vi "AlliGator Phasor Ratio Actions.vi"(0 "AlliGator Q Elements in":T4[](array[typedef]), 1 "VI in":refnum<vi>, 2 "Script in":bool, 5 "data value reference in":refnum<data-value>, 7 "AlliGator Q Event in":T5=enum."GUI:Idle", 9 "Data":variant, 11 "error in (no error)":errorcluster, 12 "AlliGator Ctrl Refnums":T6) -> (3 "Script out":bool, 4 "AlliGator Q Elements out":T4[](array[typedef]), 6 "Data Value Reference out":refnum<data-value>, 10 "[Notebook Message]":T1[](array[typedef]) {"Message Style"."Text Alignment" items=["Left", "Right", "Center"]}, 15 "error out":errorcluster)   [LabVIEW 2021, in "AlliGator Action Engine.lvlib"]
doc: "Processes AlliGator phasor ratio-related actions."
uses:
  AlliGator Action Engine.lvlib
  AlliGator Internal Variables v2.ctl
  <vilib>/vision/Image Controls.llb/IMAQ Image.ctl
  AlliGator Gate Image Set.ctl
  AlliGator FLI Dataset Type.ctl
  AlliGator Data Series Type.ctl
  AlliGator Dataset Channel.ctl
  AlliGator Gate Arithmetic.ctl
  AlliGator Displayed Image.ctl
  Image/Named ROI Description.ctl
  AlliGator Decay Metadata v3.ctl
  AlliGator Decay Background Subtraction Info.ctl
  AlliGator Baseline Subtraction Method.ctl
  Graphs/XY Graph/XY Graph Plot Shift Parameters.ctl
  Graphs/XY Graph/XY Graph Plot Shift Method.ctl
  AlliGator Decay Extrapolation Parameters.ctl
  Phasor/Calibration Phasor (m, phi).ctl
  Phasor/Phasor Reference Series.ctl
  Phasor/Phasor Calibration Map v2.ctl
  Phasor/Phasor (g, s).ctl
  AlliGator Raw Phasor Plot Data v4.ctl
  Phasor/Phasor Standard Deviation Options.ctl
  AlliGator Phasor Multi-Harmonic Data.ctl
  Phasor/Phasor Harmonic Data.ctl
  AlliGator Decay Fit Options & Parameters v2.ctl
  Fits/IRF(X)PSED/Decay Fit Options v2.ctl
  Fits/Decay Convolution/Decay Model.ctl
  Fits/Residual Type.ctl
  Fits/IRF(X)PSED/Fit Weights Type.ctl
  Fits/Non-linear Fitting Method v2.ctl
  Fits/Fit Calculation Method.ctl
  Fits/Non-linear Fitting Algorithm.ctl
  AlliGator Decay Fit Parameter Constraints 2.ctl
  Fits/IRF(X)PSED/Decay Fit Parameters In List.ctl
  Fits/IRF(X)PSED/MLE Baseline Offset Type.ctl
  AlliGator Decay Preprocessing Parameters.ctl
  Fits/IRF(X)PSED/Decay Fit Parameters & Derived Quantities List.ctl
  AlliGator Q Event.ctl
  AlliGator Ctrl Refnums.ctl
  AlliGator Other Ctrl Refnums.ctl
  AlliGator State Indicator.ctl
  AlliGator Phasor Plot Ctrl Refnums.ctl
  AlliGator Phasor Graph Ctrl Refnums.ctl
  Phasor/Phasor Calibration Type.ctl
  AlliGator Dataset Ctrl Refnums.ctl
  AlliGator Registered Events Ctrl Refnums.ctl
  AlliGator Image Histogram Control Refnums.ctl
  Histograms/Linear Histogram Options.ctl
  Histograms/Histogram Bin Option.ctl
  Histograms/Histogram Bin Position.ctl
  AlliGator Decay Fit Map Control Refnums.ctl
  AlliGator Q Element.ctl
  Notebook/Notebook Message Object.ctl
  Rich Text Box/Text Formatting.ctl
  Rich Text Box/Text Colors.ctl
  AlliGator Phasor Ratio at Mouse Location Data.ctl
  Graphs/XY Graph/XY Graph Mouse Click Event Data.ctl
  Graphs/XY Graph/XY Graph Refnum.ctl
  <vilib>/Utility/miscctls.llb/LVPoint32TypeDef.ctl
  AlliGator Phasor Reference Data.ctl
  Alligator Elements Order in Action Stack.ctl
  AlliGator State Indicators List.ctl
  AlliGator Variables List.ctl
  Variant/Variant to Data/Variant to I32.vi
  Graphs/Get Plot at Mouse Click (XY Graph)/Get Plot at Mouse Click [AAC].vi
  Variant/Variant to Data/Variant to Boolean.vi
  Variant/Variant to Data/Variant to Path.vi
  AlliGator Add Single Action to Stack.vi
  Variant/Variant to Data/Variant to DBL.vi
  Variant/Variant to Data/Variant to Data.lvlib
  GUI/GUI.lvlib
  AlliGator Source Image.lvlib
  AlliGator Phasor Graph.lvlib
  AlliGator Phasor Ratio.lvlib
  Rich Text Box/Rich Text Box.lvlib
  AlliGator Internal Variables.lvlib
  Graphs/XY Graph/XY Graph Add-Ons.lvlib
  Graphs/Graphs.lvlib
  AlliGator Globals, Variables & Constants.lvlib
  AlliGator GUI.lvlib
  AlliGator Settings.lvlib
  AlliGator Phasor Calibration.lvlib
  Notebook/Notebook.lvlib
  Phasor/Phasor.lvlib
  Image/Image.lvlib
  AlliGator Decay Preprocessing.lvlib
  AlliGator Files.lvlib
  AlliGator Phasor Plot.lvlib
  Fits/Fits.lvlib
  AlliGator Decay Fit.lvlib
  AlliGator Decay Fit Parameter Map.lvlib
  AlliGator Dual-Channel Datasets.lvlib
  Histograms/Histogram Window.lvlib
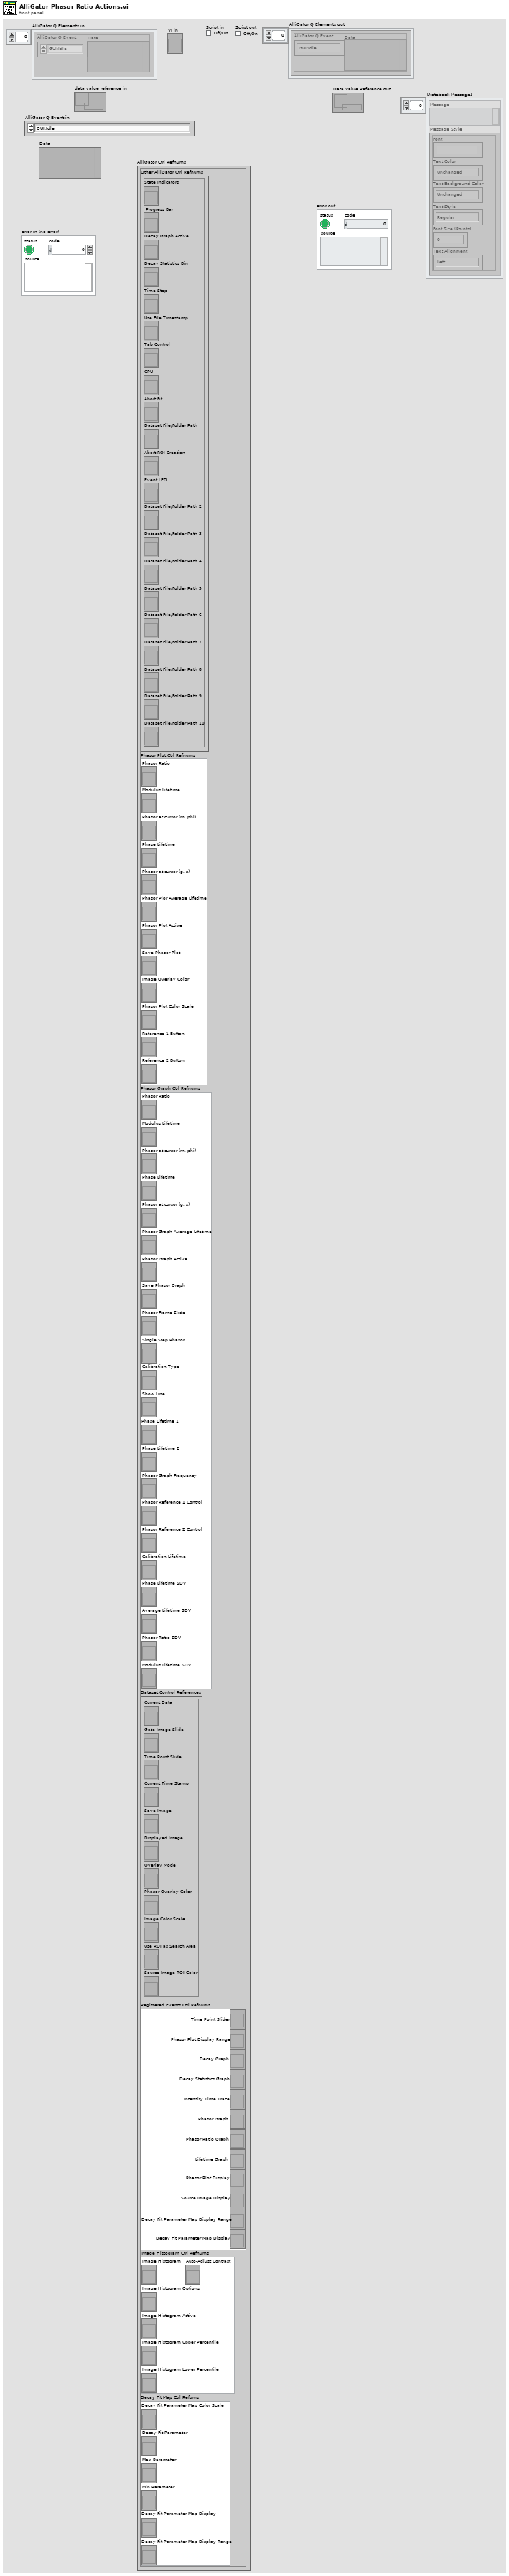
[diagram p1: front panel]
types:
  T1 = typedef "Notebook.lvlib/Notebook Message Object.ctl" = cluster{"Message":string, "Message Style":T2}
  T2 = typedef "Rich Text Box.lvlib/Text Formatting.ctl" = cluster{"Font":string, "Text Color":T3, "Text Background Color":T3, "Text Style":enum16{"Regular", "Bold", "Italic", "Underline", "Strikeout"}, "Font Size (Points)":dbl, "Text Alignment":i32}
  T3 = typedef "Rich Text Box.lvlib/Text Colors.ctl" = enum16{"Unchanged", "Black", "Blue", "Brown", "Gray", "Green", "Orange", "Pink", "Red", "White"}
  T4 = typedef "AlliGator Action Engine.lvlib/AlliGator Q Element.ctl" = cluster{"AlliGator Q Event":T5, "Data":variant}
  T5 = typedef "AlliGator Action Engine.lvlib/AlliGator Q Event.ctl" = enum16{"---- Files ----", "Files:Set Batch Export Files To Save", "Files:Set Dataset Loading & Pre-processing Options", "Files:Check #Frames in Dataset", "Files:Increment Frame Index", "Files:Open Mask Image", "Files:Open White Light Image", "Files:Open Single Dataset", "Files:New Folder of Folders Selected", "Files:Load File (all Types)_Scriptable", "Files:Move Flattened Series to Folders Series", "Files:Select Folder", "Files:Load FLI Dataset", "Files:Load Swiss SPAD 1 Dataset", "Files:Load Swiss SPAD 2 Dataset", "Files:Load .sdt FLI Dataset", "Files:Load .ptu FLI Dataset", "Files:Load .bin FLI Dataset", "Files:Load Single Gate Image Folder", "Files:Load I/m/phi Dataset (deprecated)", "Files:Load Single Image", "Files:Subtract Background File", "Files:Export FLI Dataset", "Files:Load HDF5 FLI Dataset", "Files:Set Destination File Path", "Files:Save Mask Image", "Files:Batch Conversion", "Files:New Folder Selected", "Files:Close FLI Dataset", "Files:Close FLI Dataset Series", "Files:Close White Light Image", "Files:Close Mask Image", "---- FLI Dataset ----", "FLI Dataset:Channel Arithmetic", "FLI Dataset:Export Average Lifetime Map as ASCII", "FLI Dataset:Export User-Defined Quantity Map as ASCII", "FLI Dataset:Python Function FLI Dataset Event", "FLI Dataset:ROI Analysis", "FLI Dataset:Tilted Logistic Square Gated IRF Characteristics Map", "FLI Dataset:Logistic Square Gated IRF Characteristics Map", "FLI Dataset:Square Gated IRF Characteristics Map", "FLI Dataset:Multi-ROI Single-Pixel Phasor Analysis", "FLI Dataset:Multi-ROI Single-Pixel NLSF Analysis", "FLI Dataset:All ROIs IRF Extraction", "FLI Dataset:All ROIs Decay Fit Non-Interactive (Fast + Individual IRF)", "FLI Dataset:All ROIs Phasor Analysis", "FLI Dataset:All ROIs Decay Fit", "FLI Dataset:Fluorescence Decay Statistics", "FLI Dataset:Update Decay Statistics Graph", "FLI Dataset:Get Decay from ROI", "FLI Dataset:All ROIs Average Lifetimes", "---- FLI Dataset Series ----", "FLI Dataset Series:Sum All Datasets in Series", "FLI Dataset Series:Add Dataset to Accumulated Dataset", "FLI Dataset Series:Display Accumulated Dataset", "FLI Dataset Series:Clear Dataset Series Sum", "FLI Dataset Series:Time-Series Analysis (NLSF)", "FLI Dataset Series:Time-Series Analysis (Phasor)", "---- Image ----", "Image:Update Image Profile Plots", "Image:Image Histogram Cursor Move", "Image:Image Histogram", "Image:Image Contrast", "Image:Set Image Histogram Cursor Move Flag", "Image:Clear Image Overlay", "Image:Use ROI as Search Area", "Image:Set ROI Diameter", "Image:Save Image Data as TIFF", "Image:Save Displayed Image with Overlay", "Image:Save Image Overlay Only", "Image:Save Image as Hot Pixel Mask", "Image:Change Source Image Color Palette", "Image:Copy Image to Clipboard", "Image:Source Image ROI Selection", "Image:Delete All ROIs", "Image:Delete All Unselected ROIs", "Image:Delete ROI", "Image:Merge All ROIs", "Image:Store ROI", "Image:Source Image ROI Storage", "Image:Export ROI Description to Notebook", "Image:Save ROI", "Image:Load ROI", "Image:Paste ROI Definition", "Image:Clear ROI", "Image:Identify ROIs in Mask Image", "Image:Create Complementary ROI", "Image:Create Contour ROI", "Image:Create ROI(s) from Pixels with Peak above Min_Scriptable", "Image:Create ROI(s) from Pixels with Intensity above Min_Scriptable", "Image:Compute ROI Statistics", "Image:Delete ROI(s) based on ROI Characteristics", "Image:Create ROI Grid", "Image:ROI to Individual Pixel ROIs", "Image:Python Function Source Image Event", "Image:Show Phasor Calibration Map ROI Centers", "Image:Convert ROI to Mask Image", "Image:Mouse Move", "Image:Mouse Up", "Image:Set Source Image Mouse Move Flag", "Image:Add Scale Bar Overlay", "Image:Delete Existing ROIs Option", "---- Decay ----", "Decay:Clear IRF/Reference Plot", "Decay:Clear Local IRFs", "Decay:Add Decay to Graph", "Decay:Smoothen Plot", "Decay:Smoothen Plot Tail", "Decay:Average Selected Plots", "Decay:Extract IRF", "Decay:Optimal IRF Extraction", "Decay:Threshold IRF", "Decay:Fit to Model IRF", "Decay:Fit IRF to Square Gate", "Decay:Fit IRF to Logistic Square Gate", "Decay:Fit IRF to Tilted Logistic Square Gate", "Decay:Create Bounding Cursors Set", "Decay:Export Bounding Cursors Definition to Notebook", "Decay:Denoise Plot", "Decay:Compute Cumulative Function", "Decay:Use as Reference Decay", "Decay:Show Reference Decay/IRF", "Decay:Extrapolate Decay", "Decay:Create Head & Tail Bounding Cursors", "Decay:Store Cursor-defined Head & Tail Fractions", "Decay:Rebin Plot", "Decay:1-Normalize Decay", "Decay:[0-1]-Normalize Plot", "Decay:Straighten Decay", "Decay:Shift Decay", "Decay:Fold Decay", "Decay:Fit Decay", "Decay:Global Fit of Selected Decays", "Decay:Post Global Fit Script", "Decay:Add Global Fit Parameters to Graph", "Decay:Add Decay Parameter(s) to Plot (Graph)", "Decay:Export Decay to Phasor Graph", "Decay:Plot Decay Shifts", "Decay:Compute Average Lifetime", "Decay:Plot Convolution", "Decay:Graph Tip Strip Update", "---- Decay Statistics ----", "Decay Statistics:Tip Strip Update", "---- Intensity Time Trace ----", "Intensity Time Trace:Use File Timestamp", "Intensity Time Trace:Load Intensity Corrections File", "Intensity Time Trace:Clear Intensity Corrections File", "Intensity Time Trace:Tip Strip Update", "---- Phasor Plot ----", "Phasor Plot:Build Phasor Plot", "Phasor Plot:Change Phasor Plot Color Palette", "Phasor Plot:Adjust Phasor Plot Display Range", "Phasor Plot:Highlight Image ROI in Phasor Plot", "Phasor Plot:Save Phasor Plot Image with Overlay", "Phasor Plot:Export Complex Phasor Map", "Phasor Plot:Export Phasor Ratio Map", "Phasor Plot:Export Average Lifetime Map", "Phasor Plot:Compute Phase Lifetime Histogram", "Phasor Plot:Compute Phasor Ratio Histogram", "Phasor Plot:Compute Phase Lifetime vs Intensity Scatter Plot", "Phasor Plot:Weber 2-Component Decomposition", "Phasor Plot:Update Phasor Color Map Vertices", "Phasor Plot:Clear Phasor Overlay", "Phasor Plot:Use Segment Extremities as References", "Phasor Plot:Use UC/Segment Intersections as References", "Phasor Plot:Use UC/Principal Axis Intersections as References", "Phasor Plot:Use UC/Linear Fit Intersections as References", "Phasor Plot:Update Phasor Plot Reference", "Phasor Plot:Show Local Phasor Info in Phasor Plot", "Phasor Plot:Update Phasor Plot State", "Phasor Plot:Phasor Plot ROI Storage", "Phasor Plot:Phasor Plot ROI Selection", "Phasor Plot:Python Function Phasor Plot Event", "Phasor Plot:Overlay Phasor ROI, Ratio or Map in Source Image", "Phasor Plot:Compute Decay of Selected Phasors", "Phasor Plot:Phasor at Image Pixel", "Phasor Plot:Mouse Move", "Phasor Plot:Mouse Up", "Phasor Plot:Display Range Mouse Move", "Phasor Plot:Set Mouse Move Flag", "---- Phasor Graph ----", "Phasor Graph:Calibrated Phasor Map Series", "Phasor Graph:Whole Image Phasor Scatter Plot (Todo)", "Phasor Graph:Get Phasor Value", "Phasor Graph:Create New Phasor Plot Dialog", "Phasor Graph:Update Last Phasor Value", "Phasor Graph:Update Phasor (m, phi)", "Phasor Graph:Remove Single Phasor from Plot", "Phasor Graph:Add Single Phasor to Plot", "Phasor Graph:Remove Phasor Plot", "Phasor Graph:Remove Selected Phasor Plots", "Phasor Graph:Clear Phasor Data", "Phasor Graph:Clear Phasor Graph", "Phasor Graph:Cursor Move", "Phasor Graph:Draw Cursor Connecting Line", "Phasor Graph:Clear Cursor Connecting Line", "Phasor Graph:Find UC Intersection", "Phasor Graph:Use UC/Cursor-Defined Line Intersections", "Phasor Graph:Use Selected Plots Fitted Line/UC Intersections", "Phasor Graph:Use Selected Plots Principal Axis/UC Intersections", "Phasor Graph:Show Single Phasor", "Phasor Graph:Save Single Phasor Plot", "Phasor Graph:Save All Phasor Plots", "Phasor Graph:Load Phasor Plot(s)", "Phasor Graph:Phasor Multiplication", "Phasor Graph:Compute Average Phasor", "Phasor Graph:Compute Multiple Average Phasors (Selected Plots)", "Phasor Graph:Export Single Phasor Plot Phase Lifetimes", "Phasor Graph:Phase Lifetime Trajectory", "Phasor Graph:Phase Lifetime vs Intensity Scatter Plot (deprecated)", "Phasor Graph:Parameter 2 vs Parameter 1 Scatter Plot", "Phasor Graph:Use Cursor n Location", "Phasor Graph:Set Reference n to Current Phase Lifetime Value", "Phasor Graph:Set Reference n to Lifetime Value", "Phasor Graph:Set Cursor n Location", "Phasor Graph:Save Phasor Graph Image", "Phasor Graph:Update SEPL Plot", "Phasor Graph:Export Single Phasor Plot Data", "Phasor Graph:Export Selected Phasor Plots Data", "Phasor Graph:Python Function Phasor Graph Event", "Phasor Graph:Tip Strip Update", "---- Calibration ----", "Calibration:Set Calibration Type", "Calibration:Load/Save Phasor Calibration", "Calibration:Load/Save Phasor Calibration Series", "Calibration:Load/Save Phasor Calibration Map", "Calibration:Use as Calibration", "Calibration:Compute Optimal Calibration from Phasor References", "Calibration:Clear Phasor Calibration", "Calibration:Single Phasor Calibration Information", "Calibration:Use as Calibration Series", "Calibration:Use as Calibration Map", "Calibration:Clear Calibration Series", "Calibration:Phasor Calibration Series Information", "Calibration:Clear Calibration Map", "Calibration:Phasor Calibration Map Information", "Calibration:Apply Phasor Calibration", "Calibration:Update Single Plot Calibration", "Calibration:Update Multiple Plots Calibration", "Calibration:Clear Single Plot Calibration", "Calibration:Clear All Plots Calibrations", "Calibration:Clear Plot(s) Calibration(s)?", "Calibration:Phasor Calibration Maps (# Gates Series)", "---- Phasor Ratio ----", "Phasor Ratio:Clear Reference n", "Phasor Ratio:Toggle Selected Plot(s)  Lock to Reference 1", "Phasor Ratio:Use as Reference n", "Phasor Ratio:Send Reference n to Notebook", "Phasor Ratio:Toggle Selected Plot(s)  Lock to Reference 2", "Phasor Ratio:Compute Phasor Ratio at Mouse Location", "Phasor Ratio:Compute Phasor Plot's Average Phasor Ratio", "Phasor Ratio:Compute Time-Series Phasor Ratios", "Phasor Ratio:Fit Line to Phasor Ratio Plot", "Phasor Ratio:Save References", "Phasor Ratio:Load References", "Phasor Ratio:Update Phasor Reference 1", "Phasor Ratio:Update Phasor Reference 2", "Phasor Ratio:Move Cursor n to Reference n", "Phasor Ratio:Use as Phasor Reference 1 Lifetime", "Phasor Ratio:Use as Phasor Reference 2 Lifetime", "Phasor Ratio:Export Phasor Ratio Map as ASCII", "Phasor Ratio:Tip Strip Update", "---- Lifetime & Other Parameters Graph ----", "Lifetime:Tip Strip Update", "---- Decay Fit Parameter Map ----", "Decay Fit Parameter Map:Export ROI NLSF Data as ASCII", "Decay Fit Parameter Map:Set Decay Fit  Parameter Map Selection", "Decay Fit Parameter Map:Build Decay Fit Parameter Map", "Decay Fit Parameter Map:Change Decay Fit Parameter Map Color Palette", "Decay Fit Parameter Map:Export Decay Fit Parameter Map Data as ASCII", "Decay Fit Parameter Map:Export All Decay Fit Parameter Maps Data as ASCII", "Decay Fit Parameter Map:Send Map Data to Lifetime Graph", "Decay Fit Parameter Map:Save Decay Fit Parameter Map Image", "Decay Fit Parameter Map:Save-Load IRFs & Fit Data", "Decay Fit Parameter Map:Update Local Decay Plots", "Decay Fit Parameter Map:Python Function Decay Fit Parameters Map Event", "Decay Fit Parameter Map:Overlay Decay Fit Parameter Map in Source Image", "Decay Fit Parameter Map:Plot Map Data vs Intensity", "Decay Fit Parameter Map:Mouse Up", "Decay Fit Parameter Map:Display Range Mouse Move", "---- Generic Graph ----", "Generic Graph:Generic XY Graph Event", "Generic Graph:Python Function XY Graph Event", "Generic Graph:New Plot", "Generic Graph:Save Plot", "Generic Graph:XY Plot Histogram", "Generic Graph:Set XY Graph Plot Name", "Generic Graph:Set Last Cursor Style", "Generic Graph:Tip Strip Update", "---- GUI ----", "GUI:Start Script", "GUI:Type of Displayed Image Changed", "GUI:Gate Image Slide Changed", "GUI:Show Busy Icon", "GUI:Show Busy Icon & Abort Button", "GUI:Hide Busy Icon", "GUI:Hide Busy Icon & Abort Button", "GUI:Abort", "GUI:End Script", "GUI:Start Timing", "GUI:End Timing", "GUI:Set State Indicator", "GUI:Send Parameters JSON Strings to Clipboard", "GUI:Set Gate Step", "GUI:Idle", "GUI:Initialization", "GUI:Quit", "GUI:Increment Dataset Index", "GUI:Set Dataset Index to -1", "GUI:Time Series Slider Moved", "GUI:Time Series Slider Changed", "GUI:Toggle Playback or Loop", "GUI:Playback Script", "GUI:Set Phasor Frequency", "GUI:Open Window", "GUI:Start Test Script", "GUI:End Test Script", "DEBUG"}
  T6 = typedef "AlliGator GUI.lvlib/AlliGator Ctrl Refnums.ctl" = cluster{"Other AlliGator Ctrl Refnums":T7, "Phasor Plot Ctrl Refnums":T8, "Phasor Graph Ctrl Refnums":T9, "Dataset Control References":T10, "Registered Events Ctrl Refnums":T11, "Image Histogram Ctrl Refnums":T12, "Decay Fit Map Ctrl Refums":T13}
  T7 = typedef "AlliGator GUI.lvlib/AlliGator Other Ctrl Refnums.ctl" = cluster{"State Indicators":refnum<vi>, " Progress Bar":refnum<vi>, "Decay Graph Active":refnum<vi>, "Decay Statistics Bin":refnum<vi>, "Time Step":refnum<vi>, "Use File Timestamp":refnum<vi>, "Tab Control":refnum<vi>, "CPU":refnum<vi>, "Abort Fit":refnum<vi>, "Dataset File/Folder Path":refnum<vi>, "Abort ROI Creation":refnum<vi>, "Event LED":refnum<vi>, "Dataset File/Folder Path 2":refnum<vi>, "Dataset File/Folder Path 3":refnum<vi>, "Dataset File/Folder Path 4":refnum<vi>, "Dataset File/Folder Path 5":refnum<vi>, "Dataset File/Folder Path 6":refnum<vi>, "Dataset File/Folder Path 7":refnum<vi>, "Dataset File/Folder Path 8":refnum<vi>, "Dataset File/Folder Path 9":refnum<vi>, "Dataset File/Folder Path 10":refnum<vi>}
  T8 = typedef "AlliGator GUI.lvlib/AlliGator Phasor Plot Ctrl Refnums.ctl" = cluster{"Phasor Ratio":refnum<vi>, "Modulus Lifetime":refnum<vi>, "Phasor at cursor (m, phi)":refnum<vi>, "Phase Lifetime":refnum<vi>, "Phasor at cursor (g, s)":refnum<vi>, "Phasor Plor Average Lifetime":refnum<vi>, "Phasor Plot Active":refnum<vi>, "Save Phasor Plot":refnum<vi>, "Image Overlay Color":refnum<vi>, "Phasor Plot Color Scale":refnum<vi>, "Reference 1 Button":refnum<vi>, "Reference 2 Button":refnum<vi>}
  T9 = typedef "AlliGator GUI.lvlib/AlliGator Phasor Graph Ctrl Refnums.ctl" = cluster{"Phasor Ratio":refnum<vi>, "Modulus Lifetime":refnum<vi>, "Phasor at cursor (m, phi)":refnum<vi>, "Phase Lifetime":refnum<vi>, "Phasor at cursor (g, s)":refnum<vi>, "Phasor Graph Average Lifetime":refnum<vi>, "Phasor Graph Active":refnum<vi>, "Save Phasor Graph":refnum<vi>, "Phasor Frame Slide":refnum<vi>, "Single Step Phasor":refnum<vi>, "Calibration Type":refnum<vi>, "Show Line":refnum<vi>, "Phase Lifetime 1":refnum<vi>, "Phase Lifetime 2":refnum<vi>, "Phasor Graph Frequency":refnum<vi>, "Phasor Reference 1 Control":refnum<vi>, "Phasor Reference 2 Control":refnum<vi>, "Calibration Lifetime":refnum<vi>, "Phase Lifetime SDV":refnum<vi>, "Average Lifetime SDV":refnum<vi>, "Phasor Ratio SDV":refnum<vi>, "Modulus Lifetime SDV":refnum<vi>}
  T10 = typedef "AlliGator GUI.lvlib/AlliGator Dataset Ctrl Refnums.ctl" = cluster{"Current Data":refnum<vi>, "Gate Image Slide":refnum<vi>, "Time Point Slide":refnum<vi>, "Current Time Stamp":refnum<vi>, "Save Image":refnum<vi>, "Displayed Image":refnum<vi>, "Overlay Mode":refnum<vi>, "Phasor Overlay Color":refnum<vi>, "Image Color Scale":refnum<vi>, "Use ROI as Search Area":refnum<vi>, "Source Image ROI Color":refnum<vi>}
  T11 = typedef "AlliGator GUI.lvlib/AlliGator Registered Events Ctrl Refnums.ctl" = cluster{"Time Point Slider":refnum<vi>, "Phasor Plot Display Range":refnum<vi>, "Decay Graph":refnum<vi>, "Decay Statistics Graph":refnum<vi>, "Intensity Time Trace":refnum<vi>, "Phasor Graph":refnum<vi>, "Phasor Ratio Graph":refnum<vi>, "Lifetime Graph":refnum<vi>, "Phasor Plot Display":refnum<vi>, "Source Image Display":refnum<vi>, "Decay Fit Parameter Map Display Range":refnum<vi>, "Decay Fit Parameter Map Display":refnum<vi>}
  T12 = typedef "AlliGator GUI.lvlib/AlliGator Image Histogram Control Refnums.ctl" = cluster{"Image Histogram":refnum<vi>, "Image Histogram Options":refnum<vi>, "Image Histogram Active":refnum<vi>, "Image Histogram Upper Percentile":refnum<vi>, "Image Histogram Lower Percentile":refnum<vi>, "Auto-Adjust Contrast":refnum<vi>}
  T13 = typedef "AlliGator Decay Fit Parameter Map.lvlib/AlliGator Decay Fit Map Control Refnums.ctl" = cluster{"Decay Fit Parameter Map Color Scale":refnum<vi>, "Decay Fit Parameter":refnum<vi>, "Max Parameter":refnum<vi>, "Min Parameter":refnum<vi>, "Decay Fit Parameter Map Display":refnum<vi>, "Decay Fit Parameter Map Display Range":refnum<vi>}
  T14 = typedef "AlliGator Phasor Ratio.lvlib/AlliGator Phasor Ratio at Mouse Location Data.ctl" = cluster{"Mouse Click Event Data":T15, "Interactive?":bool}
  T15 = typedef "XY Graph Add-Ons.lvlib/XY Graph Mouse Click Event Data.ctl" = cluster{"Multiplot XY Graph":T16, "Mouse Coordinates":T17}
  T16 = typedef "XY Graph Add-Ons.lvlib/XY Graph Refnum.ctl" = refnum<vi>
  T17 = typedef "LVPoint32TypeDef.ctl" = cluster{"Horizontal":i32, "Vertical":i32}
  T18 = typedef "AlliGator Phasor Ratio.lvlib/AlliGator Phasor Reference Data.ctl" = cluster{"Data Type":string, "Data":variant}
  T19 = typedef "AlliGator Action Engine.lvlib/Alligator Elements Order in Action Stack.ctl" = enum16{"Enqueue 2 AFTER 1", "Enqueue 2 BEFORE 1"}
  T20 = typedef "AlliGator Globals, Variables & Constants.lvlib/AlliGator Variables List.ctl" = enum16{"---- GUI ----", "Initialization Status", "State Indicators Refnum", "Original AlliGator Menu Items", "Current Action Loop State", "Script in progress", "Playback", "Loop Playback", "Search ROI Used", "Search ROI", "Decay Graph Max Legend Size", "Intensity Graph Max Legend Size", "Decay Statistics Graph Max Legend Size", "Phasor Graph Max Legend Size", "Phasor Ratio Graph Max Legend Size", "Lifetime Graph Max Legend Size", "---- Files ----", "Export Dataset Frames as Individual Files", "Show Batch Export Help Balloons", "Frames in Dataset", "ptu File Frame Start Indices", "Current Frame in Dataset", "Current Frame Timestamp", "------ Python Plugins ------", "Python Plugins Information", "Python Session", "Valid Python Session?", "---- Source Image ----", "Dataset Loaded", "Dataset Metadata", "Dataset Channel", "Dataset Data Description", "Background Dataset Metadata", "Background Dataset Channel", "Background Dataset Data Description", "Background File Subtraction", "Background File Path", "Background File Pile-up Correction", "Background File Pixel Well Capacity", "Background File Scaling Factor", "Source Image ROIs", "Current Source Image ROI", "Source Image ROI Event Refnum", "X_Source Image Display Range", "X_Source Image Palette Information", "Source Image Palette List", "Source Image Scale", "Current Dataset Load Settings", "Source Image:ROI Overlay Color", "---- Image Profile Window ----", "Image Profile:Overlay ROI in Source Image", "Image Profile Window Event Refnum", "Image Profile:IntensityType", "Image Profile:Intensity Average Type", "Image Profile:Intensity-weighted SDV", "Image Profile:Box Profile Type", "Image Profile Window Open", "Image Profile:Plotted Fit Parameter", "X_Type of Displayed Image", "X_Time Gate Slider", "Dataset Path", "Source Image Overlay to Erase", "Is Displayed Image Accumulated", "White Light Image Modified", "Mask Image Modified", "Macrotime Gate Separation", "------ Phasor Graph -------", "Phasor Graph:Show Line", "---- Phasor Plot ---", "Phasor Plot Parameters Changed", "FLI Dataset Modified since last Phasor Plot Calculation", "Phasor Harmonics Data", "Selected Phasor Harmonics", "Phasor Harmonic Manager Event Refnum", "Phasor Plot ROIs", "Current Phasor Plot ROI", "Phasor Plot ROI Event Refnum", "Phasor Plot Image Reference Points", "Phasor Plot Computed", "Phasor Plot Palette Information", "Phasor Plot Palette List", "Phasor Ratio Palette Information", "Phasor Ratio Palette List", "Phasor Image Scale", "Phasor Plot Image Overlay to Erase", "Phasor Plot Image Elements to Update", "Current Phasor Plot Calculation Parameters", "Current Phasor Calibration Options", "Reset Cumulated Phasor Plot", "Phasor Ratio Reference 1", "Phasor Ratio Lifetime Reference 1", "Phasor Ratio Reference 1 Frequency", "Phasor Ratio Reference 2", "Phasor Ratio Lifetime Reference 2", "Phasor Ratio Reference 2 Frequency", "---- Decay Analysis ----", "Number of Selected Decays to Fit", "LS Fit Results", "LAR Fit Results", "BS Fit Results", "Last Decay Max - Min", "Best Fit Parameters", "Best Fit Parameter Names", "Actual Size X", "Actual Size Y", "Binning X", "Binning Y", "Actual # Gates", "Dataset Number", "Gates to...", "Gates Skipped", "Gates to keep", "Gate Step", "Gate Separation", "Reversed Gates", "Pile-up Correction", "Pixel Well Capacity", "Background Subtracted", "Background Subtraction Method", "Background Definition Range", "Background File (deprecated)", "Number of Dataset Accumulated", "Array of Accumulated Dataset Paths", "Do Averaged Datasets", "Destination File Path", "Process Plot Target", "Use 1/D as Phasor Frequency", "---- Decay Fit Parameter Map -----", "Decay Fit Parameter Map Palette Information", "Decay Fit Parameter Map Palette List", "Local Decay Graph Window Event Refnum", "------- Local Decay Window ---------", "Use normalized IRF for convolution", "----- Miscellaneous ----", "Skippable Dialog Windows Status"}
  T21 = typedef "AlliGator Action Engine.lvlib/AlliGator State Indicators List.ctl" = enum16{"Phasor Calibration Defined", "Phasor Calibration Series Defined", "Phasor Calibration Map Defined", "Phasor Reference 1 Defined", "Phasor Reference 2 Defined", "Lifetime Reference 1 Defined", "Lifetime Reference 2 Defined", "Phasor Calibration Used", "Phasor Calibration Series Used", "Phasor Calibration Map Used", "Dataset Update Needed", "Phasor Plot Update Needed", "Reference/IRF Defined", "Individual IRFs Defined"}
  T22 = typedef "Phasor.lvlib/Phasor (g, s).ctl" = cluster{"g":dbl, "s":dbl}
  T23 = cluster{"Phasor Ratio Reference 1":T22, "Reference Lifetime 1":dbl[unit], "Phasor Ratio Reference 2":T22, "Reference Lifetime 2":dbl[unit]}
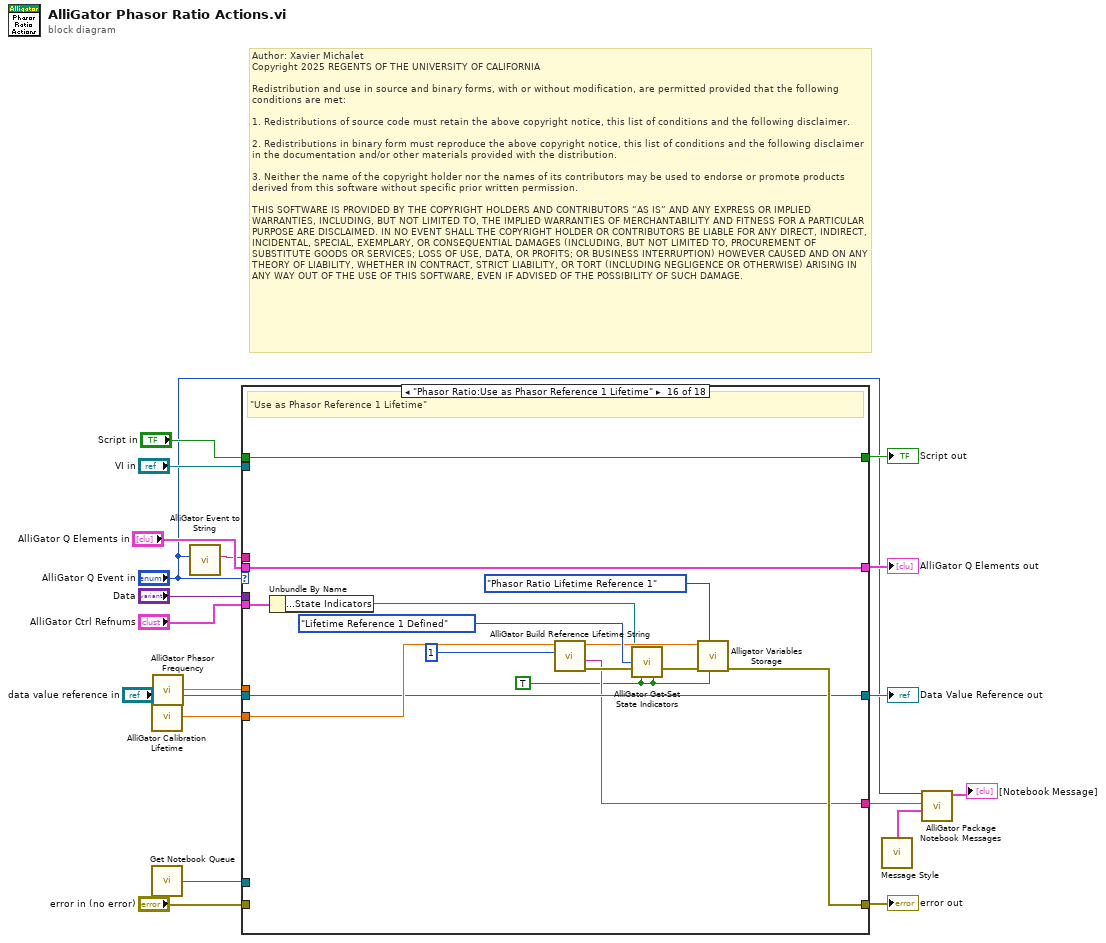
[diagram p0: block diagram]
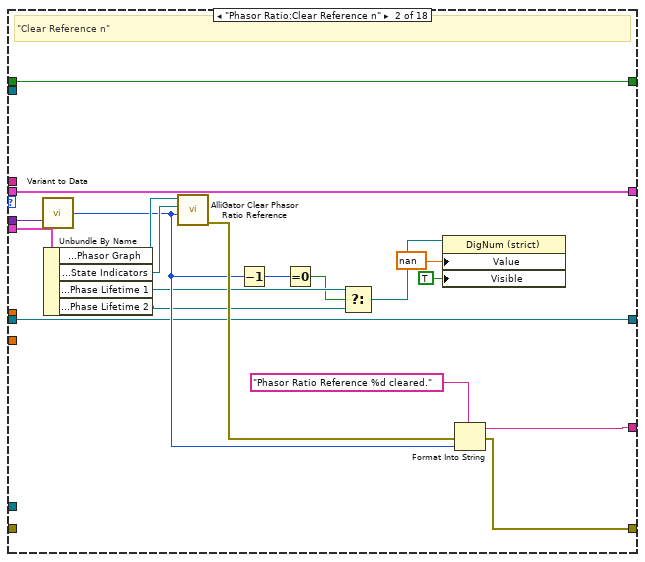
[diagram p3: hidden frame]
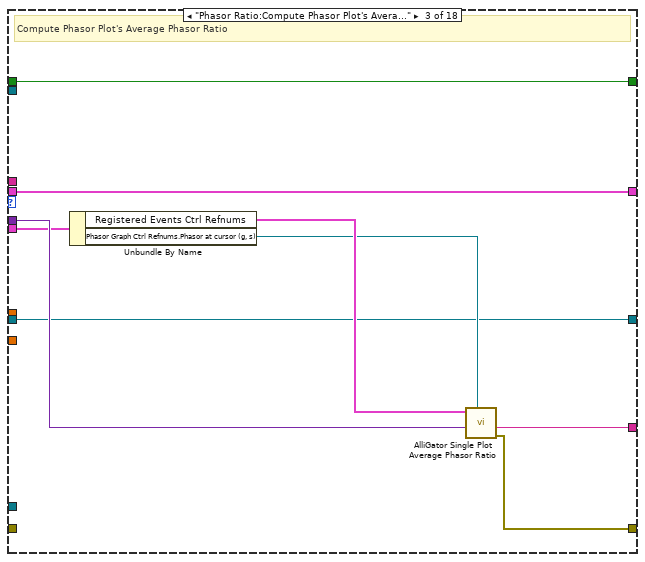
[diagram p4: hidden frame]
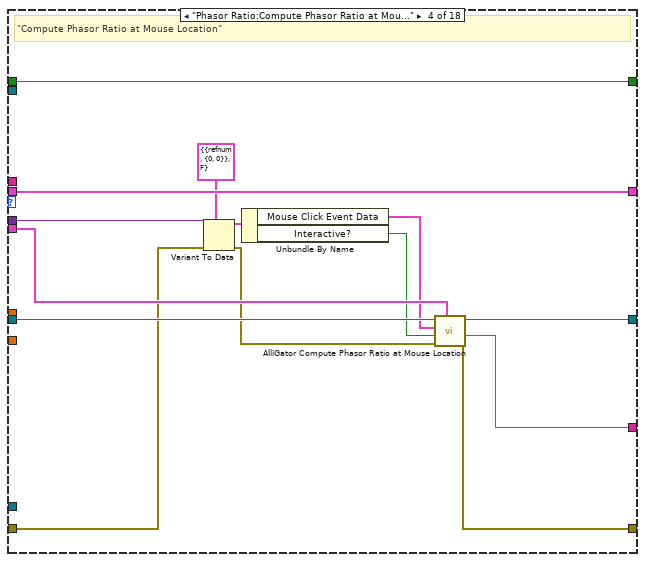
[diagram p5: hidden frame]
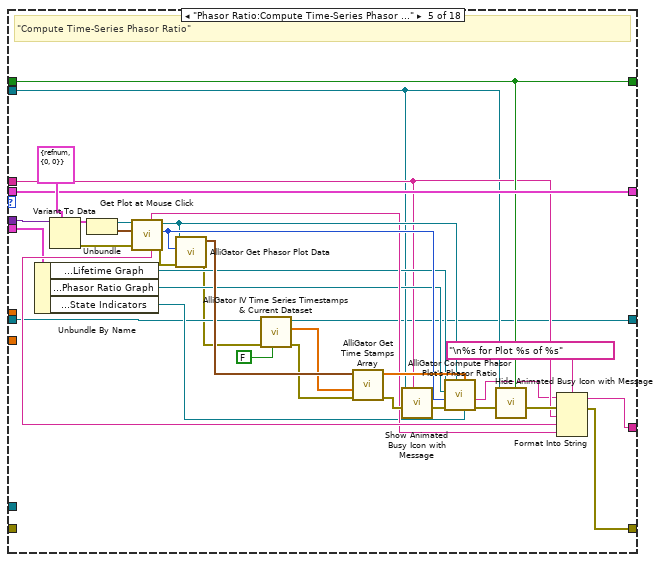
[diagram p6: hidden frame]
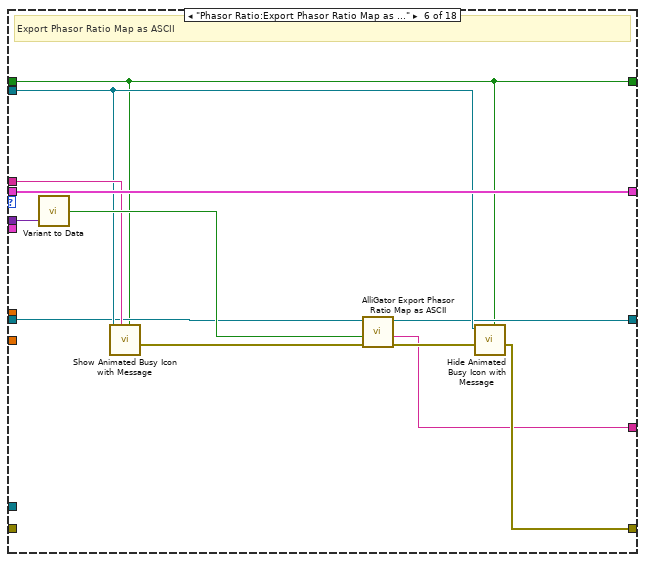
[diagram p7: hidden frame]
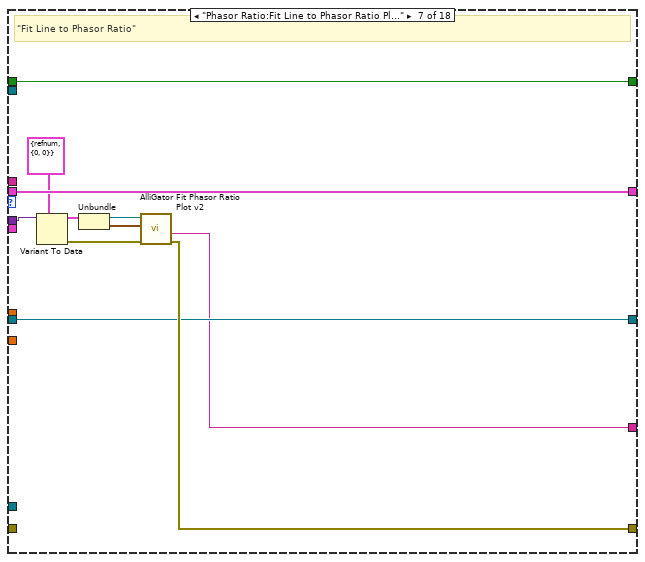
[diagram p8: hidden frame]
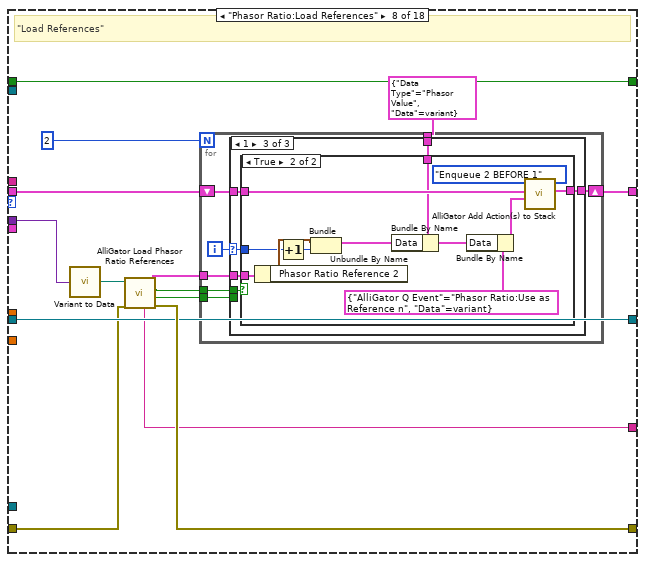
[diagram p9: hidden frame]
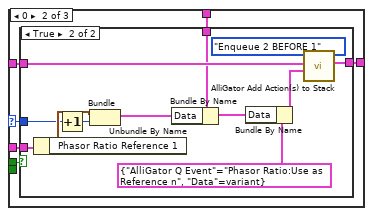
[diagram p11: hidden frame]
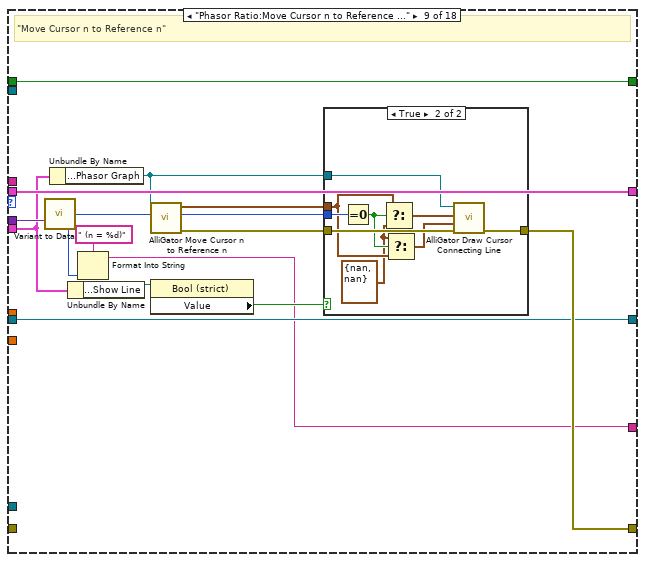
[diagram p14: hidden frame]
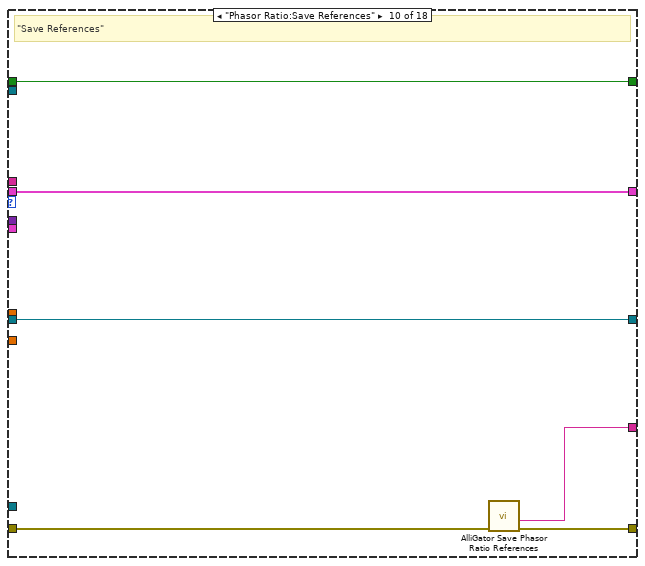
[diagram p16: hidden frame]
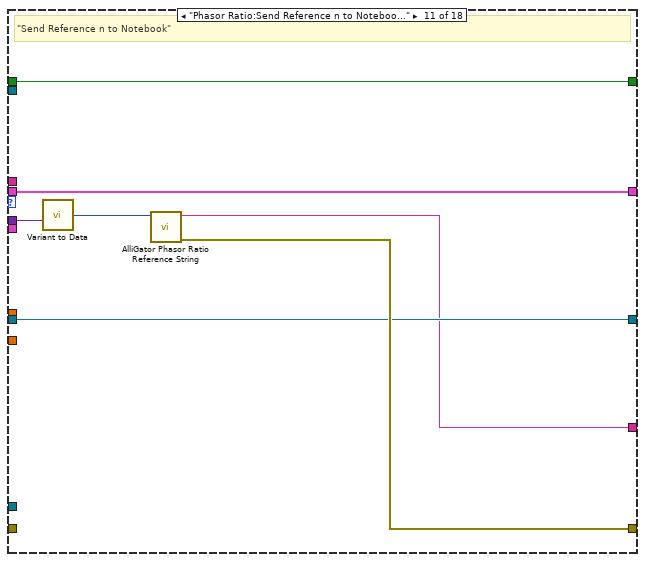
[diagram p17: hidden frame]
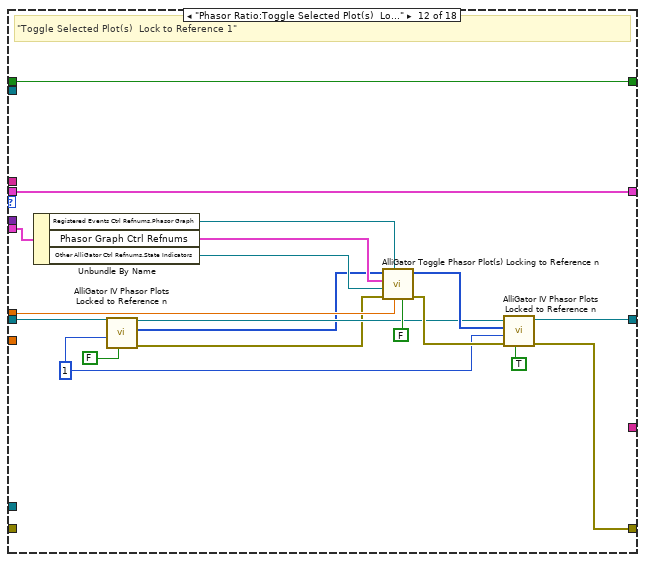
[diagram p18: hidden frame]
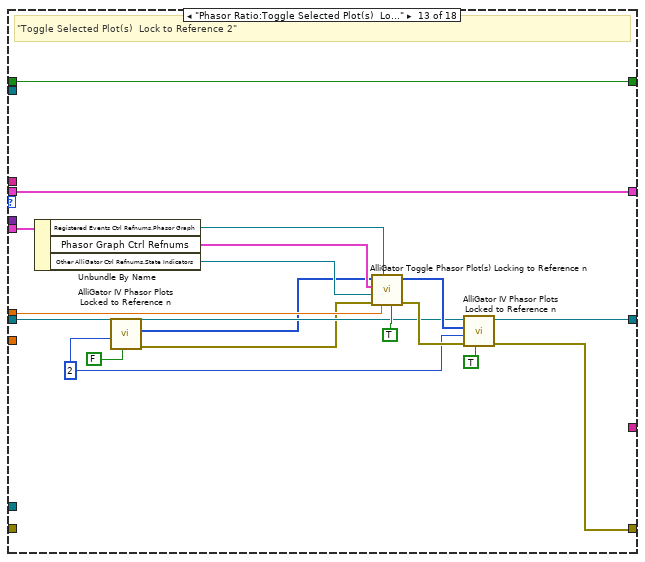
[diagram p19: hidden frame]
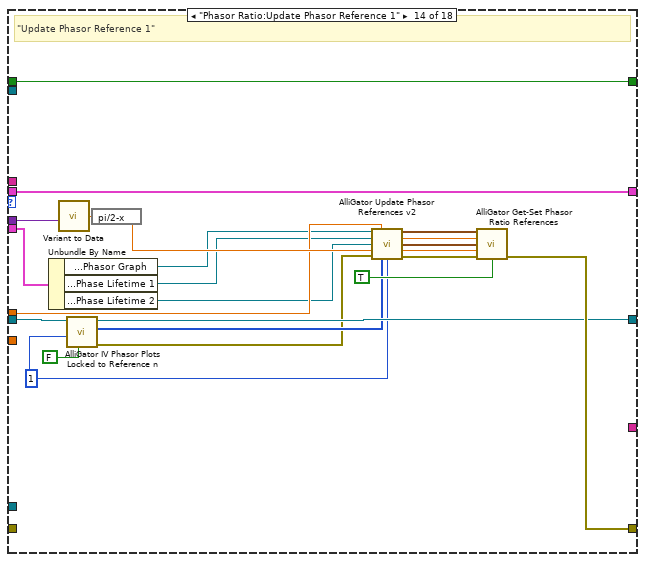
[diagram p20: hidden frame]
diagram:
  # "Author: Xavier Michalet\nCopyright 2025 REGENTS OF THE UNIVERSITY OF CALIFORNIA\n\nRedistribution and use in source and binary forms, with or without modification, are permitted provided that the following conditions are met:\n\n1. Redistributions of source code must retain the above copyright notice, this list of conditions and the following disclaimer.\n\n2. Redistributions in binary form must reproduce the above copyright notice, this list of conditions and the following disclaimer in the documentation and/or other materials provided with the distribution.\n\n3. Neither the name of the copyright holder nor the names of its contributors may be used to endorse or promote products derived from this software without specific prior written permission.\n\nTHIS SOFTWARE IS PROVIDED BY THE COPYRIGHT HOLDERS AND CONTRIBUTORS “AS IS” AND ANY EXPRESS OR IMPLIED WARRANTIES, INCLUDING, BUT NOT LIMITED TO, THE IMPLIED WARRANTIES OF MERCHANTABILITY AND FITNESS FOR A PARTICULAR PURPOSE ARE DISCLAIMED. IN NO EVENT SHALL THE COPYRIGHT HOLDER OR CONTRIBUTORS BE LIABLE FOR ANY DIRECT, INDIRECT, INCIDENTAL, SPECIAL, EXEMPLARY, OR CONSEQUENTIAL DAMAGES (INCLUDING, BUT NOT LIMITED TO, PROCUREMENT OF SUBSTITUTE GOODS OR SERVICES; LOSS OF USE, DATA, OR PROFITS; OR BUSINESS INTERRUPTION) HOWEVER CAUSED AND ON ANY THEORY OF LIABILITY, WHETHER IN CONTRACT, STRICT LIABILITY, OR TORT (INCLUDING NEGLIGENCE OR OTHERWISE) ARISING IN ANY WAY OUT OF THE USE OF THIS SOFTWARE, EVEN IF ADVISED OF THE POSSIBILITY OF SUCH DAMAGE."
  n1 = call "AlliGator Calibration Lifetime.vi"() -> ("Calibration Lifetime"=w17:dbl[unit])
  n2 = call "Get Notebook Queue.vi"() -> ("Notebook Queue"=w19:refnum<queue>)  [unwired: 9 in]
  n3 = call "AlliGator Phasor Frequency.vi"() -> ("Phasor Frequency"=w12:dbl[unit])
  n4 = call "AlliGator Event to String.vi"("AlliGator Q Event"="AlliGator Q Event in") -> ("String"=w6:string)  [unwired: 8 in]
  n5 = case shown="\"Phasor Ratio:Use as Phasor Reference 1 Lifetime\"" "AlliGator Q Event in" {
    tunnel: "Data" -> [_ w42 w49 w59 w100 w111 w122 w126 w197 _ w218 _ _ w281 w303 _ _ w360]
    tunnel: "AlliGator Q Elements in" -> [w23 w37 w51 w65 w86 w112 w123 w133 w196 w213 w220 w239 w258 w259 w304 w317 w330 w359]
    tunnel: [w23 w37 w51 w65 w86 w112 w123 w131 w196 w213 w220 w239 w258 w259 w304 w317 w330 w359] -> w8
    tunnel: "VI in" -> [_ _ _ _ w74 w107 _ _ _ _ _ _ _ _ _ _ _ w347]
    tunnel: w19 -> [_ _ _ _ _ _ _ _ _ _ _ _ _ _ _ _ _ _]
    tunnel: w12 -> [_ _ _ _ _ _ _ _ _ _ _ w238 w255 w278 w300 _ _ _]
    tunnel: [w22 w39 w50 w63 w83 w101 w115 w130 w198 w211 w219 w237 w257 w277 w299 w315 w328 w333] -> w9
    tunnel: "Script in" -> [w22 w39 w50 w63 w83 w101 w115 w130 w198 w211 w219 w237 w257 w277 w299 w315 w328 w333]
    tunnel: w6 -> [_ _ _ _ w77 w108 _ _ _ _ _ _ _ _ _ _ _ w346]
    tunnel: "error in (no error)" -> [w21 _ _ w56 _ _ _ w124 _ w208 _ _ _ _ _ _ _ _]
    tunnel: [w21 w38 w48 w64 w81 w109 w117 w137 w194 w212 w216 w230 w249 w271 w293 w312 w325 w352] -> w15
    tunnel: "AlliGator Ctrl Refnums" -> [_ w35 w47 w58 w76 _ _ _ w188 _ _ w236 w256 w268 w290 w309 w322 w348]
    tunnel: w17 -> [_ _ _ _ _ _ _ _ _ _ _ _ _ _ _ w310 w323 _]
    tunnel: "data value reference in" -> [w20 w25 w44 w62 w72 w106 w114 w128 w185 w210 w215 w226 w245 w265 w287 w307 w320 w338]
    tunnel: [w20 w25 w44 w61 w73 w105 w114 w128 w185 w210 w215 w227 w248 w264 w286 w307 w320 w334] -> w5
    tunnel: [_ w24 w43 w60 w67 w102 w113 w127 w184 w209 w214 _ _ _ _ w306 _ _] -> w4
    frame "---- Phasor Ratio ----", Default {
      # "\"---- Phasor Ratio ----\""
    }
    frame "Phasor Ratio:Clear Reference n" {
      # "\"Clear Reference n\""
      n6 = call-poly "Variant to Data.vi"("Variant"=w42) -> ("Value"=w31:i32)  [unwired: 8 in]
      n7 = Unbundle By Name(w35) -> ("Registered Events Ctrl Refnums.Phasor Graph"=w33:refnum<vi>, "Other AlliGator Ctrl Refnums.State Indicators"=w34:refnum<vi>, "Phasor Graph Ctrl Refnums.Phase Lifetime 1"=w29:refnum<vi>, "Phasor Graph Ctrl Refnums.Phase Lifetime 2"=w27:refnum<vi>)
      n8 = call "AlliGator Clear Phasor Ratio Reference.vi"("Reference Number"=w31, "State Indicators Refnum"=w34, "Phasor Graph Refnum"=w33) -> ("Error Out"=w36:errorcluster)  [unwired: 8 in]
      n9 = Decrement(x=w31) -> (x-1=w30:i32)
      n10 = Equal To 0?(x=w30) -> (x = 0?=w28:bool)
      n11 = Select(t=w29, s=w28, f=w27) -> (s? t:f=w26:refnum<vi>)
      n12 = property class="DigNum (strict)"(reference=w26, "Value"=dbl[unit] nan ("Reference Lifetime 1"), "Visible"=TRUE) -> ()  [unwired: 1 in, 2 out]
      n13 = Format Into String(format string="Phasor Ratio Reference %d cleared." ("Message"), error in=w36, w31) -> (resulting string=w24:string, error out=w38:errorcluster)  [unwired: 1 in]
    }
    frame "Phasor Ratio:Compute Phasor Plot's Average Phasor Ratio" {
      # "Compute Phasor Plot's Average Phasor Ratio"
      n14 = Unbundle By Name(w47) -> ("Registered Events Ctrl Refnums"=w46:T11, "Phasor Graph Ctrl Refnums.Phasor at cursor (g, s)"=w45:refnum<vi>)
      n15 = call "AlliGator Single Plot Average Phasor Ratio.vi"("Current Phasor Ref"=w45, "Data"=w49, "Registered Events Ctrl Refnums"=w46) -> ("Error Out"=w48:errorcluster, "Message"=w43:string)  [unwired: 7 in]
    }
    frame "Phasor Ratio:Compute Phasor Ratio at Mouse Location" {
      # "\"Compute Phasor Ratio at Mouse Location\""
      n16 = Variant To Data(error in=w56, type=T14 {"Mouse Click Event Data"={"Multiplot XY Graph"=refnum, "Mouse Coordinates"={"Horizontal"=0, "Vertical"=0}}, "Interactive?"=FALSE} ("output cluster"), Variant=w59) -> (data=w55:T14, error out=w57:errorcluster)
      n17 = Unbundle By Name(w55) -> ("Mouse Click Event Data"=w54:T15, "Interactive?"=w53:bool)
      n18 = call "AlliGator Compute Phasor Ratio at Mouse Location.vi"("AlliGator Ctrl Refnums"=w58, "error in (no error)"=w57, "Interactive?"=w53, "Mouse Click Event Data"=w54, "Data Value Reference in"=w62) -> ("error out"=w64:errorcluster, "Message"=w60:string, "Data Value Reference out"=w61:refnum<data-value>)  [unwired: 4 in]
    }
    frame "Phasor Ratio:Compute Time-Series Phasor Ratios" {
      # "\"Compute Time-Series Phasor Ratio\""
      n19 = Unbundle By Name(w76) -> ("Registered Events Ctrl Refnums.Lifetime Graph"=w79:refnum<vi>, "Registered Events Ctrl Refnums.Phasor Ratio Graph"=w78:refnum<vi>, "Other AlliGator Ctrl Refnums.State Indicators"=w75:refnum<vi>)
      n20 = Variant To Data(type=T15 {"Multiplot XY Graph"=refnum, "Mouse Coordinates"={"Horizontal"=0, "Vertical"=0}} ("Mouse Click Event Data"), Variant=w100) -> (data=w96:T15, error out=w93:errorcluster)  [unwired: 1 in]
      n21 = Unbundle(w96) -> ("Multiplot XY Graph"=w95:T16, "Mouse Coordinates"=w94:T17)
      n22 = call-poly "Get Plot at Mouse Click.vi"("error in (no error)"=w93, "Mouse Click Coordinates"=w94, "XYGraph Ref"=w95) -> ("error out"=w92:errorcluster, "Plot at Coordinates"=w90:i32, "XYGraph Ref"=w89:T16, "Plot Name"=w87:string, "Graph Name"=w80:string)  [unwired: 2 in, 2 out]
      n23 = call "AlliGator Get Phasor Plot Data.vi"("error in (no error)"=w92, "Plot Idx (-1: last)"=w90, "Phasor Graph Refnum"=w89) -> ("error out"=w70:errorcluster, "Phasor Array"=w91:T22[])  [unwired: 5 in, 2 out]
      n24 = call "AlliGator IV Time Series Timestamps & Current Dataset.vi"("Get (F)/ Set"=FALSE ("Get (F)/ Set (T)"), "error in (no error)"=w70, "AlliGator IV DVR in"=w72) -> ("error out"=w69:errorcluster, "[Time-Series Timestamps]"=w71:dbl[], "AlliGator IV DVR out"=w73:refnum<data-value>)  [unwired: 5 in, 1 out]
      n25 = call "AlliGator Get Time Stamps Array.vi"("Error In"=w69, "Dataset Series Timestamps in"=w71, "Phasor Array"=w91) -> ("Error Out"=w85:errorcluster, "Dataset Series Timestamps out"=w98:dbl[])  [unwired: 7 in]
      n26 = call "Show Animated Busy Icon with Message.vi"("Message"=w77, "Error In"=w85, "Target VI Refnum"=w74) -> ("Error Out"=w84:errorcluster)  [unwired: 8 in]
      n27 = call "AlliGator Compute Phasor Plot's Phasor Ratio.vi"("State Indicators Refnum"=w75, "Time Stamp Array"=w98, "Phasor Graph"=w89, "Error In"=w84, "Plot Idx"=w90, "Phasor Ratio Graph"=w78, "Lifetime Graph"=w79) -> ("Error Out"=w99:errorcluster, "Message"=w66:string)  [unwired: 3 in]
      n28 = call "Hide Animated Busy Icon with Message.vi"("Already active? (F)"=w83, "Error In"=w99, "Target VI reference"=w74) -> ("Error Out"=w82:errorcluster)  [unwired: 8 in]
      n29 = Format Into String(format string="\n%s for Plot %s of %s", initial string=w66, error in=w82, w77, w87, w80) -> (resulting string=w67:string, error out=w81:errorcluster)
    }
    frame "Phasor Ratio:Export Phasor Ratio Map as ASCII" {
      # "Export Phasor Ratio Map as ASCII"
      n30 = call-poly "Variant to Data.vi"("Variant"=w111) -> ("Value"=w110:bool)  [unwired: 8 in]
      n31 = call "Show Animated Busy Icon with Message.vi"("Already active? (F)"=w101, "Message"=w108, "Target VI Refnum"=w107) -> ("Error Out"=w104:errorcluster)  [unwired: 8 in]
      n32 = call "AlliGator Export Phasor Ratio Map as ASCII.vi"("error in (no error)"=w104, "Dialog?"=w110, "Data Value Reference in"=w106) -> ("error out"=w103:errorcluster, "Message"=w102:string, "Data Value Reference out"=w105:refnum<data-value>)  [unwired: 6 in]
      n33 = call "Hide Animated Busy Icon with Message.vi"("Already active? (F)"=w101, "Error In"=w103, "Target VI reference"=w107) -> ("Error Out"=w109:errorcluster)  [unwired: 8 in]
    }
    frame "Phasor Ratio:Fit Line to Phasor Ratio Plot" {
      # "\"Fit Line to Phasor Ratio\""
      n34 = Variant To Data(type=T15 {"Multiplot XY Graph"=refnum, "Mouse Coordinates"={"Horizontal"=0, "Vertical"=0}} ("Mouse Click Event Data"), Variant=w122) -> (data=w119:T15, error out=w120:errorcluster)  [unwired: 1 in]
      n35 = Unbundle(w119) -> ("Multiplot XY Graph"=w118:T16, "Mouse Coordinates"=w116:T17)
      n36 = call "AlliGator Fit Phasor Ratio Plot v2.vi"("Error In"=w120, "Mouse Coordinates"=w116, "Phasor Ratio Graph Ref"=w118) -> ("Error Out"=w117:errorcluster, "Message"=w113:string)  [unwired: 5 in, 2 out]
    }
    frame "Phasor Ratio:Load References" {
      # "\"Load References\""
      n37 = call-poly "Variant to Data.vi"("Variant"=w126) -> ("Path"=w125:path)  [unwired: 8 in]
      n38 = call "AlliGator Load Phasor Ratio References.vi"("Error In"=w124, "Reference File Path (default: Dialog)"=w125) -> ("Error Out"=w137:errorcluster, "Reference 2 Loaded"=w132:bool, "Reference 1 Loaded"=w136:bool, "Phasor References"=w135:T23, "Message"=w127:string)  [unwired: 5 in]
      n39 = for {
        N: 2 -> [_]
        tunnel: w136 -> [w142]
        tunnel: w135 -> [w144]
        shift-right: [w140] -> w131
        shift-left: w133 -> [w141]
        tunnel: w132 -> [w139]
        tunnel: T18 {"Data Type"="Phasor Value", "Data"=variant} ("Phasor Reference Data") -> [w138]
        i -> [w143]
        n40 = case shown="1" w143 {
          selector: w143 -> [_ w147 w166]
          tunnel: w144 -> [_ w151 w170]
          tunnel: w142 -> [_ w150 w169]
          tunnel: w141 -> [w145 w149 w168]
          tunnel: [w145 w148 w167] -> w140
          tunnel: w139 -> [_ _ _]
          tunnel: w138 -> [_ w146 w165]
          frame -1, Default {
          }
          frame 0 {
            n41 = case shown="True" w150 {
              tunnel: w151 -> [_ w164]
              tunnel: w149 -> [w152 w163]
              tunnel: [w152 w162] -> w148
              tunnel: w147 -> [_ w157]
              tunnel: w146 -> [_ w155]
              frame False {
              }
              frame True {
                n42 = Unbundle By Name(w164) -> ("Phasor Ratio Reference 1"=w158:T22)
                n43 = Increment(x=w157) -> (x+1=w156:i32)
                n44 = Bundle("Phasor Ratio Reference 1"=w158, w156) -> (w153:cluster{"Phasor Ratio Reference 1":T22, i32})  [unwired: 1 in]
                n45 = Bundle By Name(cluster=w155, "Data"=w153) -> (w154:T18)
                n46 = Bundle By Name(cluster=T4 {"AlliGator Q Event"=enum."Phasor Ratio:Use as Reference n", "Data"=variant} ("Alligator Atomic Action"), "Data"=w154) -> (w159:T4)
                n47 = call-poly "AlliGator Add Action(s) to Stack.vi"("Elements Order in Action Stack (Default: 2 BEFORE 1)"=Alligator_Elements_Order_in_Action_Stack."Enqueue 2 BEFORE 1", "Alligator Atomic Action"=w159, "Alligator Queue Element 1"=w163) -> ("Alligator Queue Element 1 (+ 2)"=w162:T4[])  [unwired: 7 in, 1 out]
              }
            }
          }
          frame 1 {
            n48 = case shown="True" w169 {
              tunnel: w170 -> [_ w183]
              tunnel: w168 -> [w171 w182]
              tunnel: [w171 w181] -> w167
              tunnel: w166 -> [_ w176]
              tunnel: w165 -> [_ w174]
              frame False {
              }
              frame True {
                n49 = Unbundle By Name(w183) -> ("Phasor Ratio Reference 2"=w177:T22)
                n50 = Increment(x=w176) -> (x+1=w175:i32)
                n51 = Bundle("Phasor Ratio Reference 2"=w177, w175) -> (w172:cluster{"Phasor Ratio Reference 2":T22, i32})  [unwired: 1 in]
                n52 = Bundle By Name(cluster=w174, "Data"=w172) -> (w173:T18)
                n53 = Bundle By Name(cluster=T4 {"AlliGator Q Event"=enum."Phasor Ratio:Use as Reference n", "Data"=variant} ("Alligator Atomic Action"), "Data"=w173) -> (w178:T4)
                n54 = call-poly "AlliGator Add Action(s) to Stack.vi"("Elements Order in Action Stack (Default: 2 BEFORE 1)"=Alligator_Elements_Order_in_Action_Stack."Enqueue 2 BEFORE 1", "Alligator Atomic Action"=w178, "Alligator Queue Element 1"=w182) -> ("Alligator Queue Element 1 (+ 2)"=w181:T4[])  [unwired: 7 in, 1 out]
              }
            }
          }
        }
      }
    }
    frame "Phasor Ratio:Move Cursor n to Reference n" {
      # "\"Move Cursor n to Reference n\""
      n55 = call-poly "Variant to Data.vi"("Variant"=w197) -> ("Value"=w190:i32)  [unwired: 8 in]
      n56 = Unbundle By Name(w188) -> ("Registered Events Ctrl Refnums.Phasor Graph"=w193:refnum<vi>)
      n57 = Unbundle By Name(w188) -> ("Phasor Graph Ctrl Refnums.Show Line"=w187:refnum<vi>)
      n58 = Format Into String(format string=" (n = %d)", w190) -> (resulting string=w184:string)  [unwired: 2 in, 1 out]
      n59 = call "AlliGator Move Cursor n to Reference n.vi"("Reference n"=w190, "Phasor Graph Refnum"=w193) -> ("Error Out"=w195:errorcluster, "Reference Idx"=w191:i32, "Reference Phasor"=w192:T22)  [unwired: 7 in]
      n60 = property class="Bool (strict)"(reference=w187) -> ("Value"=w186:bool)  [unwired: 1 in, 2 out]
      n61 = case shown="True" w186 {
        tunnel: w193 -> [_ w207]
        tunnel: [_ w206] -> w194
        tunnel: w195 -> [_ w205]
        tunnel: w192 -> [_ w201]
        tunnel: w191 -> [_ w204]
        frame False {
        }
        frame True {
          w200 = cluster{"X":dbl, "Y":dbl} {"X"=nan, "Y"=nan} ("Reference 2")
          n62 = Equal To 0?(x=w204) -> (x = 0?=w202:bool)
          n63 = Select(t=w201, s=w202, f=w200) -> (s? t:f=w203:T22)
          n64 = Select(t=w200, s=w202, f=w201) -> (s? t:f=w199:T22)
          n65 = call "AlliGator Draw Cursor Connecting Line.vi"("Error In"=w205, "Reference 2"=w199, "Reference 1"=w203, "Phasor Graph Refnum"=w207) -> ("Error Out"=w206:errorcluster)  [unwired: 7 in]
        }
      }
    }
    frame "Phasor Ratio:Save References" {
      # "\"Save References\""
      n66 = call "AlliGator Save Phasor Ratio References.vi"("Error In"=w208) -> ("Error Out"=w212:errorcluster, "Message"=w209:string)  [unwired: 9 in]
    }
    frame "Phasor Ratio:Send Reference n to Notebook" {
      # "\"Send Reference n to Notebook\""
      n67 = call-poly "Variant to Data.vi"("Variant"=w218) -> ("Value"=w217:i32)  [unwired: 8 in]
      n68 = call "AlliGator Phasor Ratio Reference String.vi"("Reference #"=w217) -> ("Error Out"=w216:errorcluster, "Message"=w214:string)  [unwired: 9 in]
    }
    frame "Phasor Ratio:Toggle Selected Plot(s)  Lock to Reference 1" {
      w223 = 1 ("Reference n")
      # "\"Toggle Selected Plot(s)  Lock to Reference 1\""
      n69 = Unbundle By Name(w236) -> ("Registered Events Ctrl Refnums.Phasor Graph"=w232:refnum<vi>, "Phasor Graph Ctrl Refnums"=w235:T9, "Other AlliGator Ctrl Refnums.State Indicators"=w234:refnum<vi>)
      n70 = call "AlliGator IV Phasor Plots Locked to Reference n.vi"("Get (F)/ Set (T)"=FALSE, "Reference n"=w223, "AlliGator IV DVR in"=w226) -> ("error out"=w221:errorcluster, "[Phasor Plot(s) locked to Ref n"=w224:i32[], "AlliGator IV DVR out"=w225:refnum<data-value>)  [unwired: 6 in]
      n71 = call "AlliGator Toggle Phasor Plot(s) Locking to Reference n.vi"("Ref 1(F)/Ref 2(T)"=FALSE, "Phasor Frequency"=w238, "Phasor Graph Refnum"=w232, "error in"=w221, "State Indicators"=w234, "Phasor Graph Ctrl Refnums"=w235, "[Phasor Plot(s) locked to Ref n] in"=w224) -> ("error out"=w231:errorcluster, "[Phasor Plot(s) locked to Ref n] out"=w229:i32[])  [unwired: 3 in]
      n72 = call "AlliGator IV Phasor Plots Locked to Reference n.vi"("Get (F)/ Set (T)"=TRUE, "error in (no error)"=w231, "Reference n"=w223, "[Phasor Plot(s) locked to Ref n"=w229, "AlliGator IV DVR in"=w225) -> ("error out"=w230:errorcluster, "AlliGator IV DVR out"=w227:refnum<data-value>)  [unwired: 4 in, 1 out]
    }
    frame "Phasor Ratio:Toggle Selected Plot(s)  Lock to Reference 2" {
      w241 = 2 ("Reference n")
      # "\"Toggle Selected Plot(s)  Lock to Reference 2\""
      n73 = Unbundle By Name(w256) -> ("Registered Events Ctrl Refnums.Phasor Graph"=w251:refnum<vi>, "Phasor Graph Ctrl Refnums"=w254:T9, "Other AlliGator Ctrl Refnums.State Indicators"=w253:refnum<vi>)
      n74 = call "AlliGator IV Phasor Plots Locked to Reference n.vi"("Get (F)/ Set (T)"=FALSE, "Reference n"=w241, "AlliGator IV DVR in"=w245) -> ("error out"=w243:errorcluster, "[Phasor Plot(s) locked to Ref n"=w242:i32[], "AlliGator IV DVR out"=w244:refnum<data-value>)  [unwired: 6 in]
      n75 = call "AlliGator Toggle Phasor Plot(s) Locking to Reference n.vi"("Ref 1(F)/Ref 2(T)"=TRUE, "Phasor Frequency"=w255, "Phasor Graph Refnum"=w251, "error in"=w243, "State Indicators"=w253, "Phasor Graph Ctrl Refnums"=w254, "[Phasor Plot(s) locked to Ref n] in"=w242) -> ("error out"=w250:errorcluster, "[Phasor Plot(s) locked to Ref n] out"=w247:i32[])  [unwired: 3 in]
      n76 = call "AlliGator IV Phasor Plots Locked to Reference n.vi"("Get (F)/ Set (T)"=TRUE, "error in (no error)"=w250, "Reference n"=w241, "[Phasor Plot(s) locked to Ref n"=w247, "AlliGator IV DVR in"=w244) -> ("error out"=w249:errorcluster, "AlliGator IV DVR out"=w248:refnum<data-value>)  [unwired: 4 in, 1 out]
    }
    frame "Phasor Ratio:Update Phasor Reference 1" {
      w260 = 1 ("Reference n")
      # "\"Update Phasor Reference 1\""
      n77 = Unbundle By Name(w268) -> ("Registered Events Ctrl Refnums.Phasor Graph"=w269:refnum<vi>, "Phasor Graph Ctrl Refnums.Phase Lifetime 1"=w267:refnum<vi>, "Phasor Graph Ctrl Refnums.Phase Lifetime 2"=w266:refnum<vi>)
      n78 = call-poly "Variant to Data.vi"("Variant"=w281) -> ("Value"=w280:dbl)  [unwired: 8 in]
      n79 = call "AlliGator IV Phasor Plots Locked to Reference n.vi"("Get (F)/ Set (T)"=FALSE, "Reference n"=w260, "AlliGator IV DVR in"=w265) -> ("error out"=w262:errorcluster, "[Phasor Plot(s) locked to Ref n"=w263:i32[], "AlliGator IV DVR out"=w264:refnum<data-value>)  [unwired: 6 in]
      n80 = expression code="pi/2-x"(w280) -> (w279:dbl)
      n81 = call "AlliGator Update Phasor References v2.vi"("XYGraph in"=w269, "Phasor Frequency"=w278, "Phase Lifetime 1"=w267, "Phase Lifetime 2"=w266, "New Reference Phase"=w279, "Error In"=w262, "Locked Plots"=w263, "Updated Reference ID"=w260) -> ("Reference Phasor 1"=w276:T22, "Reference Lifetime 1"=w275:dbl[unit], "Reference Phasor 2"=w274:T22, "Reference Lifetime 2"=w273:dbl[unit], "Error Out"=w272:errorcluster)  [unwired: 3 in]
      n82 = call "AlliGator Get-Set Phasor Ratio References.vi"("Reference Phasor 1"=w276, "Reference Lifetime 1"=w275, "Reference Phasor 2"=w274, "Reference Lifetime 2"=w273, "error in (no error)"=w272, "Get(F)/Set"=TRUE) -> ("error out"=w271:errorcluster)  [unwired: 2 in, 7 out]
    }
    frame "Phasor Ratio:Update Phasor Reference 2" {
      w284 = 2 ("Updated Reference ID")
      # "\"Update Phasor Reference 2\""
      n83 = call-poly "Variant to Data.vi"("Variant"=w303) -> ("Value"=w302:dbl)  [unwired: 8 in]
      n84 = Unbundle By Name(w290) -> ("Registered Events Ctrl Refnums.Phasor Graph"=w291:refnum<vi>, "Phasor Graph Ctrl Refnums.Phase Lifetime 1"=w289:refnum<vi>, "Phasor Graph Ctrl Refnums.Phase Lifetime 2"=w288:refnum<vi>)
      n85 = call "AlliGator IV Phasor Plots Locked to Reference n.vi"("Get (F)/ Set (T)"=FALSE, "Reference n"=w284, "AlliGator IV DVR in"=w287) -> ("error out"=w282:errorcluster, "[Phasor Plot(s) locked to Ref n"=w285:i32[], "AlliGator IV DVR out"=w286:refnum<data-value>)  [unwired: 6 in]
      n86 = expression code="pi/2-x"(w302) -> (w301:dbl)
      n87 = call "AlliGator Update Phasor References v2.vi"("XYGraph in"=w291, "Phasor Frequency"=w300, "Phase Lifetime 1"=w289, "Phase Lifetime 2"=w288, "New Reference Phase"=w301, "Error In"=w282, "Locked Plots"=w285, "Updated Reference ID"=w284) -> ("Reference Phasor 1"=w298:T22, "Reference Lifetime 1"=w297:dbl[unit], "Reference Phasor 2"=w296:T22, "Reference Lifetime 2"=w295:dbl[unit], "Error Out"=w294:errorcluster)  [unwired: 3 in]
      n88 = call "AlliGator Get-Set Phasor Ratio References.vi"("Reference Phasor 1"=w298, "Reference Lifetime 1"=w297, "Reference Phasor 2"=w296, "Reference Lifetime 2"=w295, "error in (no error)"=w294, "Get(F)/Set"=TRUE) -> ("error out"=w293:errorcluster)  [unwired: 2 in, 7 out]
    }
    frame "Phasor Ratio:Use as Phasor Reference 1 Lifetime" {
      w305 = TRUE ("Set (T)/Unset (F)")
      # "\"Use as Phasor Reference 1 Lifetime\""
      n89 = Unbundle By Name(w309) -> ("Other AlliGator Ctrl Refnums.State Indicators"=w308:refnum<vi>)
      n90 = call "AlliGator Build Reference Lifetime String.vi"("Reference #"=1, "Lifetime"=w310) -> ("Error Out"=w314:errorcluster, "Message"=w306:string)  [unwired: 8 in]
      n91 = call "AlliGator Get-Set State Indicators.vi"("State Indicators Refnum"=w308, "AlliGator State Indicators List"=AlliGator_State_Indicators_List."Lifetime Reference 1 Defined" ("Time-Gated Phasor Analysis Task List"), "Error In"=w314, "ON/OFF"=w305, "Set (T)/Get"=w305) -> ("Error Out"=w313:errorcluster)  [unwired: 8 in, 2 out]
      n92 = call "Alligator Variables Storage.vi"("Get(F)/Set"=w305, "AlliGator Variable"=AlliGator_Variables_List."Phasor Ratio Lifetime Reference 1" ("Alligator Variable"), "Error In"=w313, "Data in"=w310) -> ("Error Out"=w312:errorcluster)  [unwired: 5 in, 2 out]
    }
    frame "Phasor Ratio:Use as Phasor Reference 2 Lifetime" {
      w319 = TRUE ("Set (T)/Unset (F)")
      # "\"Use as Phasor Reference 2 Lifetime\""
      n93 = Unbundle By Name(w322) -> ("Other AlliGator Ctrl Refnums.State Indicators"=w321:refnum<vi>)
      n94 = call "AlliGator Build Reference Lifetime String.vi"("Reference #"=2, "Lifetime"=w323) -> ("Error Out"=w327:errorcluster)  [unwired: 8 in, 1 out]
      n95 = call "AlliGator Get-Set State Indicators.vi"("State Indicators Refnum"=w321, "AlliGator State Indicators List"=AlliGator_State_Indicators_List."Lifetime Reference 2 Defined" ("Time-Gated Phasor Analysis Task List"), "Error In"=w327, "ON/OFF"=w319, "Set (T)/Get"=w319) -> ("Error Out"=w326:errorcluster)  [unwired: 8 in, 2 out]
      n96 = call "Alligator Variables Storage.vi"("Get(F)/Set"=w319, "AlliGator Variable"=AlliGator_Variables_List."Phasor Ratio Lifetime Reference 2" ("Alligator Variable"), "Error In"=w326, "Data in"=w323) -> ("Error Out"=w325:errorcluster)  [unwired: 5 in, 2 out]
    }
    frame "Phasor Ratio:Use as Reference n" {
      # "\"Use as Reference n\""
      n97 = call "AlliGator IV Last Calibrated Phasor.vi"("Get (F)/ Set (T)"=FALSE, "AlliGator IV DVR in"=w338) -> ("error out"=w336:errorcluster, "Last Calibrated Phasor"=w337:T22, "AlliGator IV DVR out"=w334:refnum<data-value>)  [unwired: 7 in]
      n98 = Unbundle By Name(w348) -> ("Other AlliGator Ctrl Refnums.State Indicators"=w350:refnum<vi>, "Registered Events Ctrl Refnums.Phasor Graph"=w358:refnum<vi>, "Phasor Graph Ctrl Refnums"=w349:T9)
      n99 = call "Show Animated Busy Icon with Message.vi"("Already active? (F)"=w333, "Message"=w346, "Error In"=w336, "Target VI Refnum"=w347) -> ("Error Out"=w353:errorcluster)  [unwired: 7 in]
      n100 = Unbundle By Name(w348) -> ("Phasor Graph Ctrl Refnums.Phase Lifetime 1"=w341:refnum<vi>, "Phasor Graph Ctrl Refnums.Phase Lifetime 2"=w340:refnum<vi>)
      n101 = call "AlliGator Get Phasor Ratio Reference v2.vi"("Error In"=w353, "Last Phasor"=w337, "Data"=w360) -> ("error out"=w357:errorcluster, "Reference #"=w344:i32, "Reference Phasor"=w351:T22)  [unwired: 6 in]
      n102 = Decrement(x=w344) -> (x-1=w343:i32)
      n103 = Equal To 0?(x=w343) -> (x = 0?=w342:bool)
      n104 = call "AlliGator Update Phasor Graph Information at Cursor.vi"("Valid?"=TRUE, "Error In"=w357, "Phasor"=w351, "Current Phasor Information Indicators"=w349) -> ("Error Out"=w356:errorcluster, "Phase Lifetime"=w354:dbl[unit])  [unwired: 6 in]
      n105 = Select(t=w341, s=w342, f=w340) -> (s? t:f=w339:refnum<vi>)
      n106 = call "AlliGator Set Phasor Reference.vi"("Lifetime"=w354, "State Indicators Refnum"=w350, "error in (no error)"=w356, "Reference Number"=w344, "Plot Data Point"=w351, "Phasor Graph Refnum"=w358) -> ("Error Out"=w355:errorcluster)  [unwired: 5 in]
      n107 = property class="DigNum (strict)"(reference=w339, "Value"=w354, "Visible"=TRUE) -> ()  [unwired: 1 in, 2 out]
      n108 = call "Hide Animated Busy Icon with Message.vi"("Already active? (F)"=w333, "Error In"=w355, "Target VI reference"=w347) -> ("Error Out"=w352:errorcluster)  [unwired: 8 in]
    }
  }
  "Data Value Reference out" <- w5
  "error out" <- w15
  "Script out" <- w9
  "AlliGator Q Elements out" <- w8
  n109 = call "Message Style.vi"() -> ("Message Formatting"=w2:T2)
  n110 = call "AlliGator Package Notebook Messages.vi"("Message Formatting"=w2, "Message"=w4, "AlliGator Q Event in"="AlliGator Q Event in") -> ("[Notebook Message]"=→"[Notebook Message]":T1[])  [unwired: 8 in]
